vi "Host_SetParameters_Thresholds.vi"(11 "Set Min/Max Values":string[](array[string])) -> (3 "Data":T1={"cRIO Data"={"HallEffect Right (cm)"=0.0, "HallEffect Left (cm)"=0.0, "Optical Sensor 1 (V)"=0.0, "Optical Sensor 2 (V)"=0.0, "24V Voltage  (V)"=0.0, "24V Current (A)"=0.0, "Contactor H1 Continuity"=0.0, "Contactor L1 Continuity "=0.0, "Contactor H2 Continuity"=0.0, "Contactor L2 Continuity "=0.0, "Time (ms)"=0.0, "Displacement (ft)"=0.0, "Velocity (ft/s)"=0.0, "ABS Pressure 1 (psig)"=0.0, "ABS Pressure 2 (psig) "=0.0, "24V Temp   (C)"=0.0, "Brake PT(psig)"=0.0, "Tank PT(psig) "=0.0, "Pump PT(psig)"=0.0, "24 Temp Average(C) "=0.0, "High Voltage 1"=FALSE}, "IMU Data"={"x acceleration (g)"=0.0, "Pressure (psia)"=0.0, "Temperature (F)"=0.0}, "BMS Data"={"Max Cell Voltage (V)"=0.0, "Max Cell ID"=0.0, "Min Cell Voltage (V)"=0.0, "Min Cell ID"=0.0, "State of Charge (%)"=0.0, "Average Voltage (V)"=0.0, "Voltage Delta (V)"=0.0, "Pack Current (A)"=0.0, "Pack Voltage (V)"=0.0, "Max Resistance (Ohm)"=0.0, "Min Resistance (Ohm)"=0.0, "Average Resistance (Ohm)"=0.0, "Delta Resistance (Ohm)"=0.0, "Highest Temperature(F)"=0.0, "BmsStatus"={"isFault"=FALSE, "isolationMonitoring"=FALSE}}, "Motor Data"={" Velocity (RPM)"=0.0, " MotorTemp(C)"=0.0, " ControlTemp(C)"=0.0, " DcLinkVolt(V)"=0.0, " ErrorCode"=0.0, "IsAlive"=FALSE, "motorStatus"={"isReady"=FALSE, "isOn"=FALSE, "isOperEn"=FALSE, "isFault"=FALSE, "isVoltEn"=FALSE, "targetReached"=FALSE, "isWarning"=FALSE}, "motorControllerState"=1}} {"Motor Data"."motorControllerState" items=["unknown"=1, "boot-up"=0, "stopped"=4, "operational"=5, "pre-operational"=127, "connection lost"=128]})   [LabVIEW 2018]
uses:
  Type_Def/TypeDef_BMSData.ctl
  Type_Def/TypeDef_cRIOData.ctl
  Type_Def/Master_DataControl.ctl
  Type_Def/TypeDef FixedMotorData.ctl
  Type_Def/TypeDef_BmsStatus.ctl
  Type_Def/Type_Def IMUData.ctl
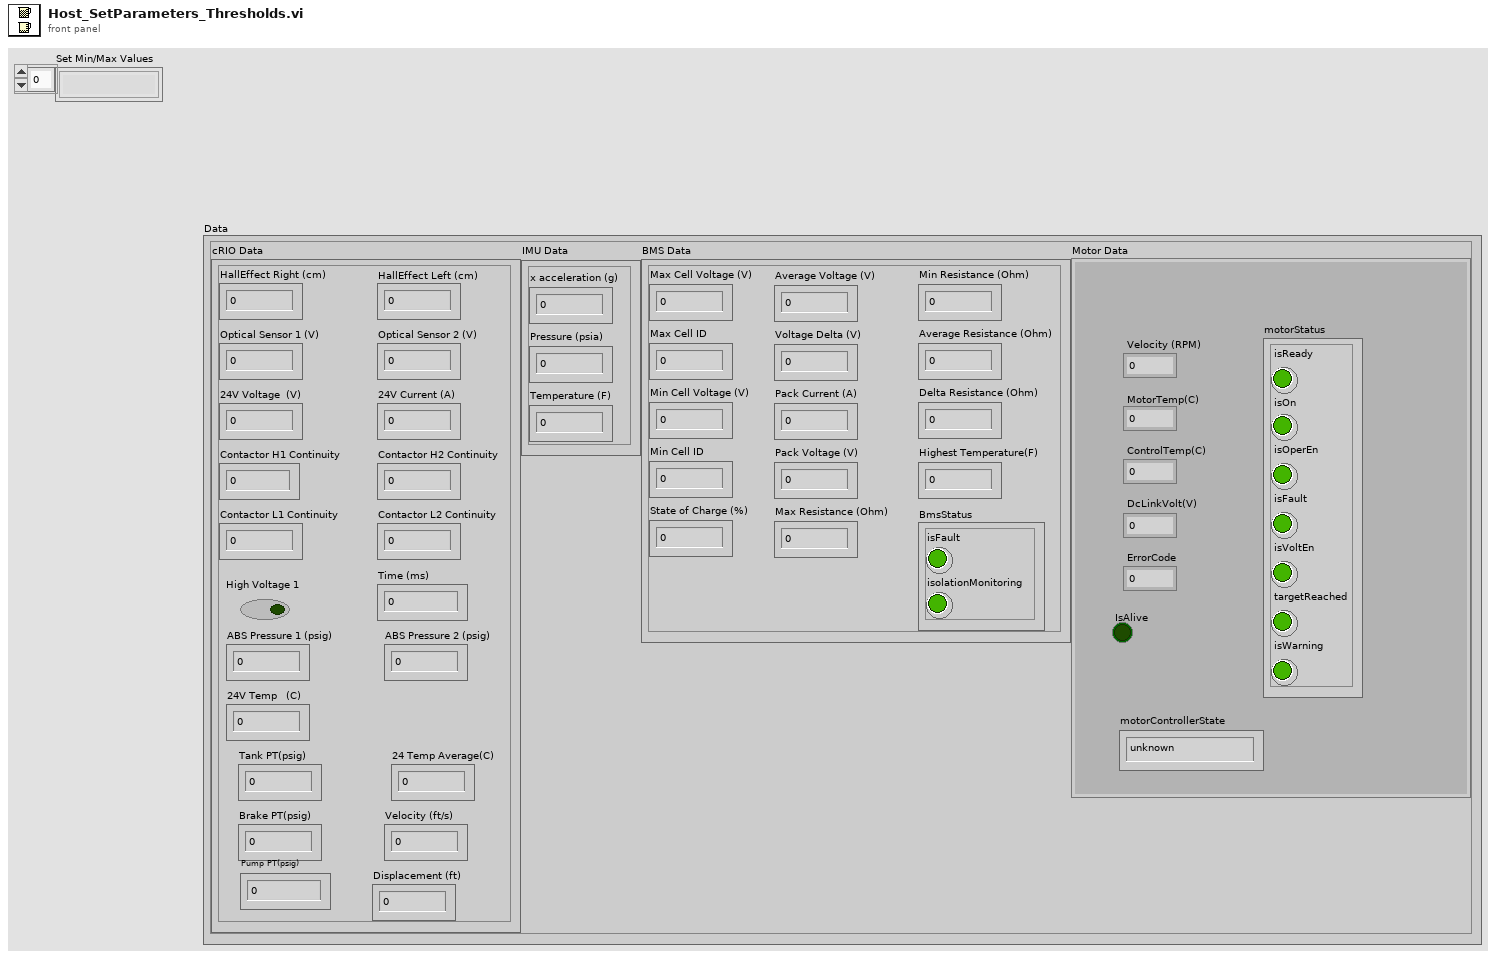
[diagram p1: front panel]
types:
  T1 = typedef "Master_DataControl.ctl" = cluster{"cRIO Data":T2, "IMU Data":T3, "BMS Data":T4, "Motor Data":T6}
  T2 = typedef "TypeDef_cRIOData.ctl" = cluster{"HallEffect Right (cm)":dbl, "HallEffect Left (cm)":dbl, "Optical Sensor 1 (V)":dbl, "Optical Sensor 2 (V)":dbl, "24V Voltage  (V)":dbl, "24V Current (A)":dbl, "Contactor H1 Continuity":dbl, "Contactor L1 Continuity ":dbl, "Contactor H2 Continuity":dbl, "Contactor L2 Continuity ":dbl, "Time (ms)":dbl, "Displacement (ft)":dbl, "Velocity (ft/s)":dbl, "ABS Pressure 1 (psig)":dbl, "ABS Pressure 2 (psig) ":dbl, "24V Temp   (C)":dbl, "Brake PT(psig)":dbl, "Tank PT(psig) ":dbl, "Pump PT(psig)":dbl, "24 Temp Average(C) ":dbl, "High Voltage 1":bool}
  T3 = typedef "Type_Def IMUData.ctl" = cluster{"x acceleration (g)":dbl, "Pressure (psia)":dbl, "Temperature (F)":dbl}
  T4 = typedef "TypeDef_BMSData.ctl" = cluster{"Max Cell Voltage (V)":dbl, "Max Cell ID":dbl, "Min Cell Voltage (V)":dbl, "Min Cell ID":dbl, "State of Charge (%)":dbl, "Average Voltage (V)":dbl, "Voltage Delta (V)":dbl, "Pack Current (A)":dbl, "Pack Voltage (V)":dbl, "Max Resistance (Ohm)":dbl, "Min Resistance (Ohm)":dbl, "Average Resistance (Ohm)":dbl, "Delta Resistance (Ohm)":dbl, "Highest Temperature(F)":dbl, "BmsStatus":T5}
  T5 = typedef "TypeDef_BmsStatus.ctl" = cluster{"isFault":bool, "isolationMonitoring":bool}
  T6 = typedef "TypeDef FixedMotorData.ctl" = cluster{" Velocity (RPM)":dbl, " MotorTemp(C)":dbl, " ControlTemp(C)":dbl, " DcLinkVolt(V)":dbl, " ErrorCode":dbl, "IsAlive":bool, "motorStatus":cluster{"isReady":bool, "isOn":bool, "isOperEn":bool, "isFault":bool, "isVoltEn":bool, "targetReached":bool, "isWarning":bool}, "motorControllerState":u16}
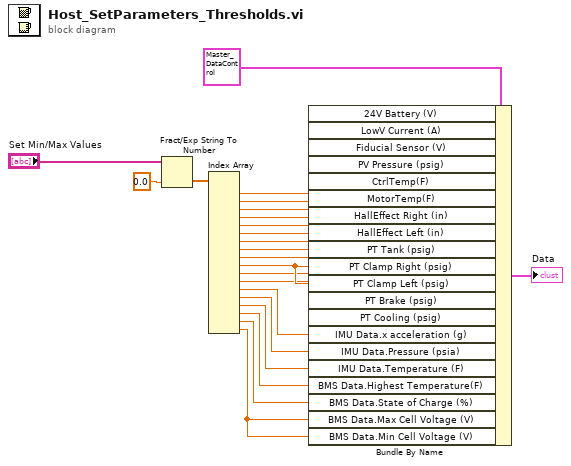
[diagram p0: block diagram]
diagram:
  n1 = Fract/Exp String To Number(string="Set Min/Max Values", default (0 dbl)=0.0 ("default (0 I32)")) -> (number=w17:dbl[])  [unwired: 2 in, 1 out]
  n2 = Index Array(array=w17) -> (element #1=w19:dbl, element #2=w20:dbl, element #3=w21:dbl, element #4=w22:dbl, element #5=w14:dbl, element #6=w13:dbl, element #7=w12:dbl, element #8=w11:dbl, element #9=w10:dbl, element #10=w9:dbl, element #11=w8:dbl, element #12=w7:dbl, element #13=w6:dbl, element #14=w5:dbl, element #15=w4:dbl, element #16=w3:dbl, element #17=w2:dbl, element #18=w1:dbl)  [unwired: 18 in]
  n3 = Bundle By Name(cluster=T1 {"cRIO Data"={"HallEffect Right (cm)"=0.0, "HallEffect Left (cm)"=0.0, "Optical Sensor 1 (V)"=0.0, "Optical Sensor 2 (V)"=0.0, "24V Voltage  (V)"=0.0, "24V Current (A)"=0.0, "Contactor H1 Continuity"=0.0, "Contactor L1 Continuity "=0.0, "Contactor H2 Continuity"=0.0, "Contactor L2 Continuity "=0.0, "Time (ms)"=0.0, "Displacement (ft)"=0.0, "Velocity (ft/s)"=0.0, "ABS Pressure 1 (psig)"=0.0, "ABS Pressure 2 (psig) "=0.0, "24V Temp   (C)"=0.0, "Brake PT(psig)"=0.0, "Tank PT(psig) "=0.0, "Pump PT(psig)"=0.0, "24 Temp Average(C) "=0.0, "High Voltage 1"=FALSE}, "IMU Data"={"x acceleration (g)"=0.0, "Pressure (psia)"=0.0, "Temperature (F)"=0.0}, "BMS Data"={"Max Cell Voltage (V)"=0.0, "Max Cell ID"=0.0, "Min Cell Voltage (V)"=0.0, "Min Cell ID"=0.0, "State of Charge (%)"=0.0, "Average Voltage (V)"=0.0, "Voltage Delta (V)"=0.0, "Pack Current (A)"=0.0, "Pack Voltage (V)"=0.0, "Max Resistance (Ohm)"=0.0, "Min Resistance (Ohm)"=0.0, "Average Resistance (Ohm)"=0.0, "Delta Resistance (Ohm)"=0.0, "Highest Temperature(F)"=0.0, "BmsStatus"={"isFault"=FALSE, "isolationMonitoring"=FALSE}}, "Motor Data"={" Velocity (RPM)"=0.0, " MotorTemp(C)"=0.0, " ControlTemp(C)"=0.0, " DcLinkVolt(V)"=0.0, " ErrorCode"=0.0, "IsAlive"=FALSE, "motorStatus"={"isReady"=FALSE, "isOn"=FALSE, "isOperEn"=FALSE, "isFault"=FALSE, "isVoltEn"=FALSE, "targetReached"=FALSE, "isWarning"=FALSE}, "motorControllerState"=1}} ("Data"), "24V Battery (V)"=w19, "LowV Current (A)"=w20, "Fiducial Sensor (V)"=w21, "PV Pressure (psig)"=w22, "CtrlTemp(F)"=w14, "MotorTemp(F)"=w13, "HallEffect Right (in)"=w12, "HallEffect Left (in)"=w11, "PT Tank (psig)"=w10, "PT Clamp Right (psig)"=w9, "PT Clamp Left (psig)"=w9, "PT Brake (psig)"=w8, "PT Cooling (psig)"=w7, "IMU Data.x acceleration (g)"=w6, "IMU Data.Pressure (psia)"=w5, "IMU Data.Temperature (F)"=w4, "BMS Data.Highest Temperature(F)"=w3, "BMS Data.State of Charge (%)"=w2, "BMS Data.Max Cell Voltage (V)"=w1, "BMS Data.Min Cell Voltage (V)"=w1) -> (→"Data":T1)
